vi "TTA_MATLAB_Generate_Report.vi"(8 "error in":errorcluster) -> (0 "error out":errorcluster)   [LabVIEW 2016]
uses:
  TTA_Globals/Test_Environment.vi
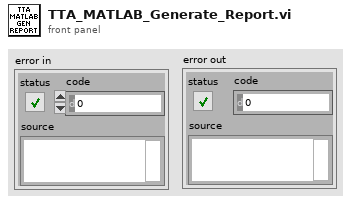
[diagram p1: front panel]
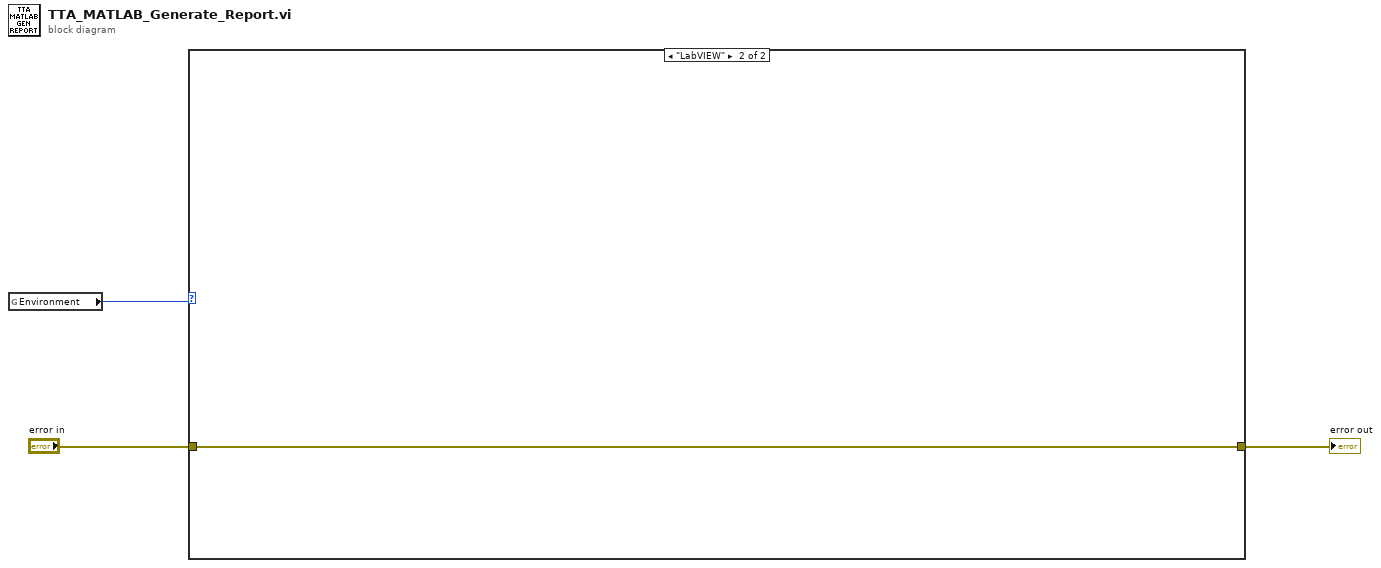
[diagram p0: block diagram]
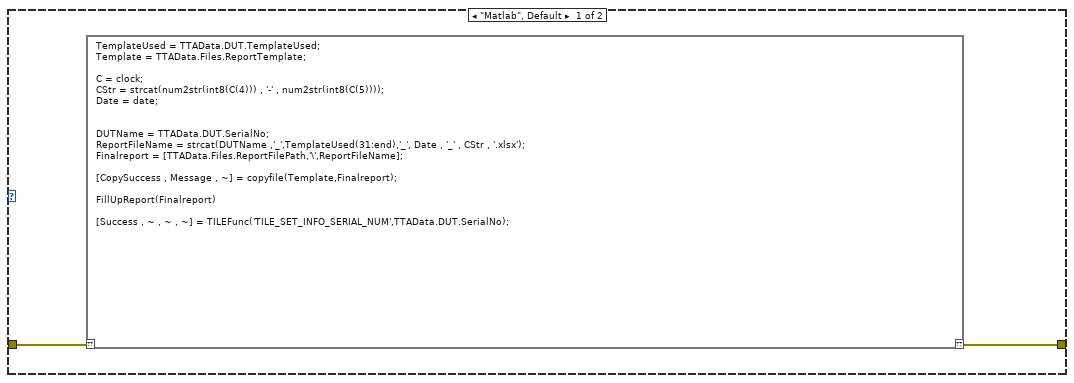
[diagram p2: hidden frame]
diagram:
  n1 = global read "Test_Environment.vi" "Environment"() -> (w1:enum16{"Matlab", "LabVIEW"})
  n2 = case shown="\"LabVIEW\"" w1 {
    tunnel: "error in" -> [w5 w6]
    tunnel: [w4 w6] -> w2
    frame "Matlab", Default {
      n3 = script code="TemplateUsed = TTAData.DUT.TemplateUsed;\nTemplate = TTAData.Files.ReportTemplate;\n\nC = clock;\nCStr = strcat(num2str(int8(C(4))) , '-' , num2str(int8(C(5))));\nDate = date;\n\n\nDUTName = TTAData.DUT.SerialNo;\nReportFileName = strcat(DUTName ,'_',TemplateUsed(31:end),'_', Date , '_' , CStr , '.xlsx');\nFinalreport = [TTAData.Files.ReportFilePath,'\\',ReportFileName];\n\n[CopySuccess , Message , ~] = copyfile(Template,Finalreport);\n\nFillUpReport(Finalreport)\n\n[Success , ~ , ~ , ~] = TILEFunc('TILE_SET_INFO_SERIAL_NUM',TTAData.DUT.SerialNo);"("??"=w5) -> ("??"=w4:errorcluster)
    }
    frame "LabVIEW" {
    }
  }
  "error out" <- w2
